vi "Web Service Settings Store.vi"(8 "error in (no error)":errorcluster, 10 "new settings":T1, 11 "action":u16(ring) items=["Initialize Settings Store", "Destroy Settings Store", "Set Settings", "Get Settings"]) -> (0 "error out":errorcluster, 2 "settings out":T1)   [LabVIEW 2020, in "CSM WebService.lvlib"]
doc: "Stores and provides access to settings used by the web service. This VI uses a functional global variable to provide access for both the weather simulator application and the web service included with the application. Because it is non-reentrant and reserved by the main application VI, the data is available throughout the application."
uses:
  CSM WebService.lvlib
  Web Service Settings.ctl
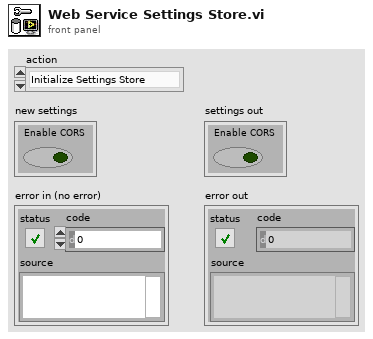
[diagram p1: front panel]
types:
  T1 = typedef "CSM WebService.lvlib/Web Service Settings.ctl" = cluster{"Enable CORS":bool}
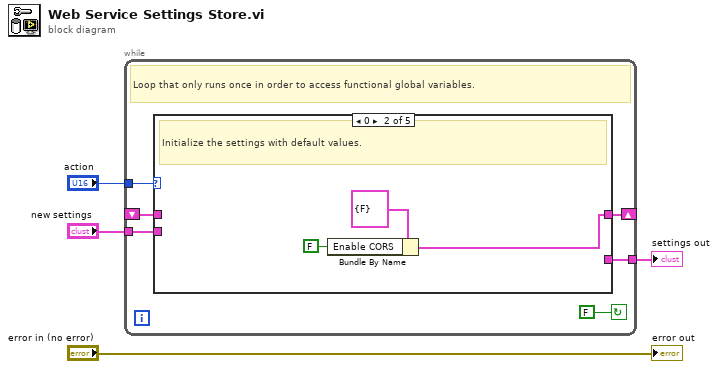
[diagram p0: block diagram]
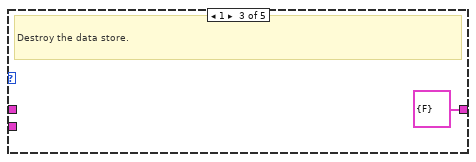
[diagram p3: hidden frame]
diagram:
  n1 = while {
    tunnel: "action" -> [w10]
    shift-right: [w8] -> _
    shift-left: _ -> [w7]
    tunnel: "new settings" -> [w6]
    tunnel: [w5] -> w2
    stop <- FALSE continue-if-true
    # "Loop that only runs once in order to access functional global variables."
    n2 = case shown="0" w10 {
      tunnel: [w11 w12 T1 {"Enable CORS"=FALSE} ("Web Service Settings") w16 w17] -> w8
      tunnel: w7 -> [w11 _ _ _ w17]
      tunnel: w6 -> [_ _ _ w16 _]
      tunnel: [_ _ _ _ w17] -> w5
      frame Default {
        # "Invalid action."
      }
      frame 0 {
        # "Initialize the settings with default values."
        n3 = Bundle By Name(cluster=T1 {"Enable CORS"=FALSE} ("Web Service Settings"), "Enable CORS"=FALSE) -> (w12:T1)
      }
      frame 1 {
        # "Destroy the data store."
      }
      frame 2 {
        # "Update the stored settings."
      }
      frame 3 {
        # "Return the stored settings."
      }
    }
  }
  "settings out" <- w2
  "error out" <- "error in (no error)"
